vi "Scalar Settings.vi"(6 "Action":T2, 8 "error in (no error)":errorcluster, 10 "Scalar Settings":T1, 11 "Item Ref":T3 format="%.0x") -> (0 "error out":errorcluster, 2 "Scalar Settings":T1, 3 "Item Ref out":T3=18446744073709551615 format="%.0x")   [LabVIEW 2019, in "FPGA Addon Shared.lvlib"]
uses:
  FPGA Addon Shared.lvlib
  <vilib>/NI VeriStand/Custom Device API/Custom Device Item Ref.ctl
  Types/FG Action.ctl
  Types/Scalar Settings.ctl
  Constants.vi
  <vilib>/NI VeriStand/Custom Device API/Get Item Property (U32).vi
  <vilib>/NI VeriStand/Custom Device API/Set Item Property (U32).vi
  <vilib>/NI VeriStand/Custom Device API/Custom Device API.lvlib
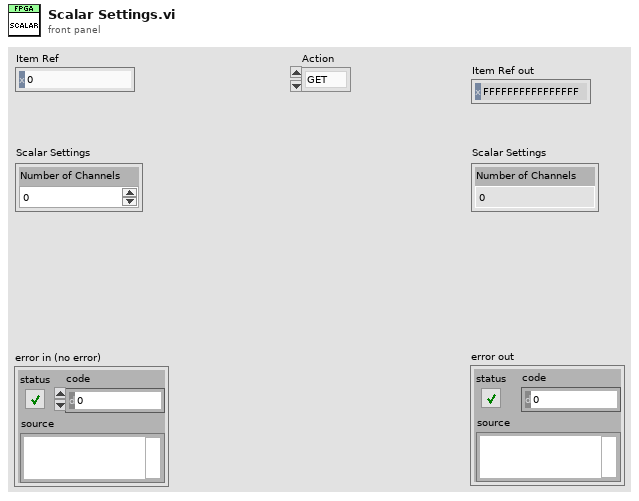
[diagram p1: front panel]
types:
  T1 = typedef "FPGA Addon Shared.lvlib/Scalar Settings.ctl" = cluster{"Number of Channels":u8}
  T2 = typedef "FPGA Addon Shared.lvlib/FG Action.ctl" = enum8{"GET", "SET"}
  T3 = typedef "Custom Device API.lvlib/Custom Device Item Ref.ctl" = u64
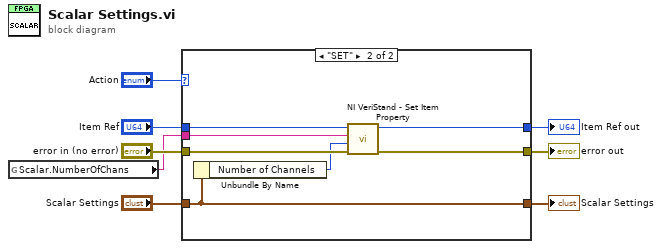
[diagram p0: block diagram]
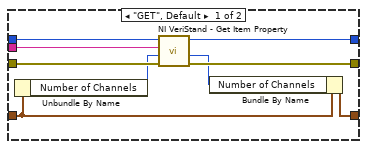
[diagram p2: hidden frame]
diagram:
  n1 = global read "Constants.vi" "Scalar.NumberOfChans"() -> (w3:string)
  n2 = case shown="\"SET\"" "Action" {
    tunnel: "error in (no error)" -> [w17 w24]
    tunnel: "Item Ref" -> [w16 w23]
    tunnel: "Scalar Settings" -> [w10 w20]
    tunnel: [w15 w22] -> w8
    tunnel: [w14 w21] -> w5
    tunnel: [w9 w20] -> w2
    tunnel: w3 -> [w13 w19]
    frame "GET", Default {
      n3 = Unbundle By Name(w10) -> ("Number of Channels"=w12:u8)
      n4 = call-poly <vilib>:"NI VeriStand - Get Item Property.vi"("error in (no error)"=w17, "Default Value"=w12, "Property Name"=w13, "Item Ref in"=w16) -> ("error out"=w15:errorcluster, "Value"=w11:u32, "Item Ref out"=w14:T3)  [unwired: 4 in, 1 out]
      n5 = Bundle By Name(cluster=w10, "Number of Channels"=w11) -> (w9:T1)
    }
    frame "SET" {
      n6 = Unbundle By Name(w20) -> ("Number of Channels"=w18:u8)
      n7 = call-poly <vilib>:"NI VeriStand - Set Item Property.vi"("error in (no error)"=w24, "Value"=w18, "Property Name"=w19, "Item Ref in"=w23) -> ("error out"=w22:errorcluster, "Item Ref out"=w21:T3)  [unwired: 5 in, 1 out]
    }
  }
  "error out" <- w8
  "Item Ref out" <- w5
  "Scalar Settings" <- w2
